vi "SetPropertyNative.vi"(8 "error in (no error)":errorcluster, 10 "Numeric":dbl, 11 "reference in":refnum<class "G#MethodTemplates.lvclass">) -> (0 "error out":errorcluster, 3 "reference out":refnum<class "G#MethodTemplates.lvclass">)   [LabVIEW 2017, in "G#MethodTemplates.lvclass"]
uses:
  <vilib>/addons/_AddQ/G#Templates/G#MethodTemplates/G#MethodTemplates.lvclass
  <vilib>/addons/_AddQ/G#Templates/G#MethodTemplates/G#MethodTemplates.lvclass/G#MethodTemplates.ctl
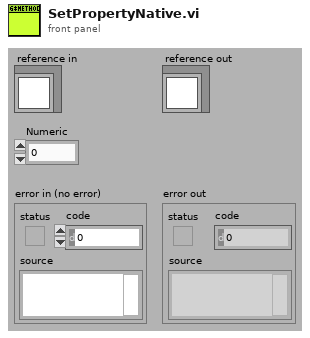
[diagram p1: front panel]
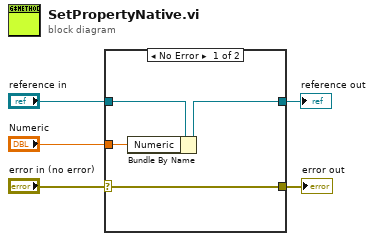
[diagram p0: block diagram]
diagram:
  n1 = case shown="No Error" "error in (no error)" {
    selector: "error in (no error)" -> [w6 w11]
    tunnel: [w6 w11] -> w4
    tunnel: [w8 w10] -> w2
    tunnel: "reference in" -> [w9 w10]
    tunnel: "Numeric" -> [w7 _]
    frame No Error {
      n2 = Bundle By Name(cluster=w9, "Numeric"=w7) -> (w8:refnum<class "G#MethodTemplates.lvclass">)
    }
    frame Error {
    }
  }
  "error out" <- w4
  "reference out" <- w2
